vi "inject_error.vi"(8 "error in":errorcluster, 10 "s":bool) -> (0 "error out":errorcluster)   [LabVIEW 2017]
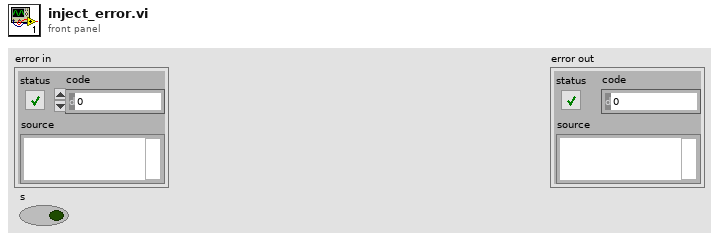
[diagram p1: front panel]
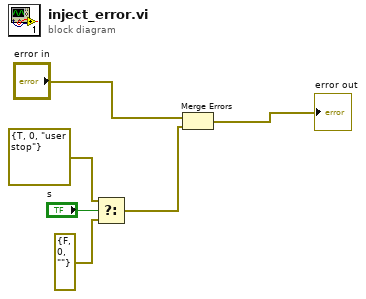
[diagram p0: block diagram]
diagram:
  n1 = Select(t=errorcluster {"status"=TRUE, "code"=0, "source"="user stop"} ("error constant"), s="s", f=errorcluster {"status"=FALSE, "code"=0, "source"=""} ("error constant")) -> (s? t:f=w1:errorcluster)
  n2 = Merge Errors("error in", w1) -> (→"error out":errorcluster)
